vi "TPNT_CheckFileSize.vi"(8 "error in (no error)":errorcluster, 10 "maxfilesize":u32, 11 "File":path) -> (0 "error out":errorcluster, 2 "file moved":bool)   [LabVIEW 2016]
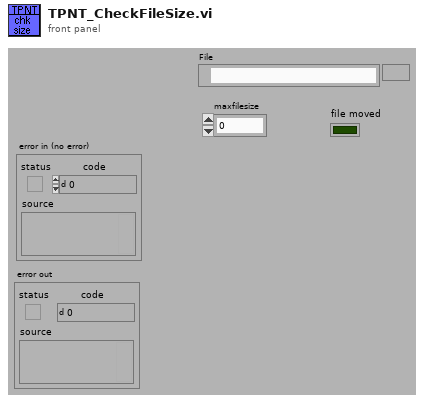
[diagram p1: front panel]
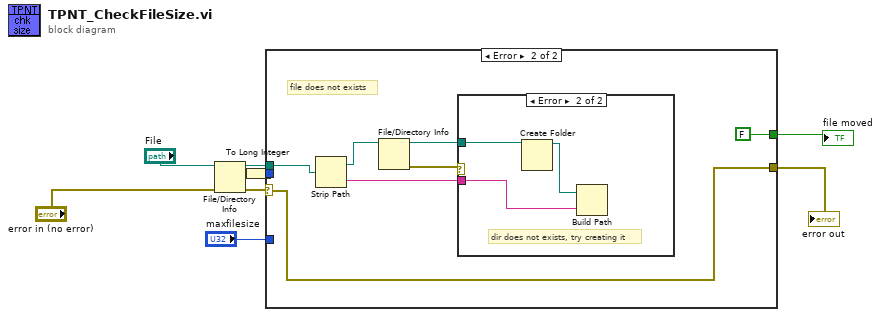
[diagram p0: block diagram]
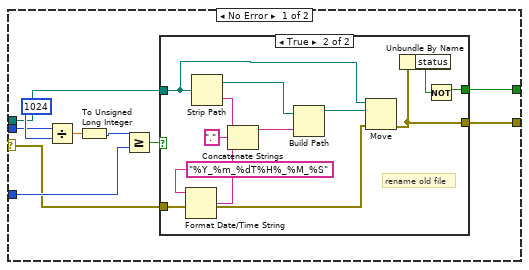
[diagram p2: hidden frame]
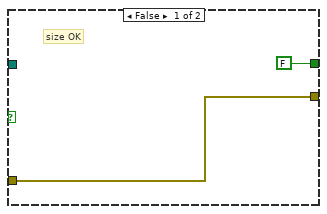
[diagram p3: hidden frame]
diagram:
  n1 = File/Directory Info(path="File", error in="error in (no error)") -> (path out=w5:path, size=w1:i64, error out=w4:errorcluster)  [unwired: 4 out]
  n2 = To Long Integer(number=w1) -> (32bit integer=w7:i32)
  n3 = case shown="Error" w4 {
    selector: w4 -> [w11 w34]
    tunnel: "maxfilesize" -> [w19 _]
    tunnel: w7 -> [w16 _]
    tunnel: w5 -> [w14 w39]
    tunnel: [w12 w34] -> w3
    tunnel: [w10 FALSE ("f")] -> w2
    frame No Error {
      n4 = Divide(x=w16, y=1024) -> (x/y=w17:dbl)
      n5 = To Unsigned Long Integer(number=w17) -> (unsigned 32bit integer=w15:u32)
      n6 = Greater Or Equal?(x=w15, y=w19) -> (x >= y?=w13:bool)
      n7 = case shown="True" w13 {
        tunnel: w14 -> [_ w26]
        tunnel: [w21 w24] -> w12
        tunnel: w11 -> [w21 w27]
        tunnel: [FALSE ("f") w22] -> w10
        frame False {
          # "size OK"
        }
        frame True {
          # "rename old file"
          n8 = Format Date/Time String(time format string (%c)="%Y_%m_%dT%H%_%M_%S") -> (date/time string=w30:string)  [unwired: 2 out]
          n9 = Strip Path(path=w26) -> (stripped path=w25:path, name=w33:string)
          n10 = Concatenate Strings(w33, "." ("string"), w30) -> (w29:string)
          n11 = Build Path(base path=w25, name or relative path=w29) -> (appended path=w28:path)
          n12 = Move(source path=w26, error in=w27, 10:w28) -> (error out=w24:errorcluster)  [unwired: 4 out]
          n13 = Unbundle By Name(w24) -> ("status"=w23:bool)
          n14 = Not(x=w23) -> (.not. x?=w22:bool)
        }
      }
    }
    frame Error {
      # "file does not exists"
      n15 = Strip Path(path=w39) -> (stripped path=w37:path, name=w38:string)
      n16 = File/Directory Info(path=w37) -> (path out=w35:path, error out=w36:errorcluster)  [unwired: 1 in, 5 out]
      n17 = case shown="Error" w36 {
        tunnel: w38 -> [_ w42]
        tunnel: w35 -> [_ w41]
        frame No Error {
          # "but directory does"
        }
        frame Error {
          # "dir does not exists, try creating it"
          n18 = Create Folder(path (use dialog)=w41) -> (created path=w43:path)  [unwired: 1 in, 3 out]
          n19 = Build Path(base path=w43, name or relative path=w42) -> ()  [unwired: 1 out]
        }
      }
    }
  }
  "error out" <- w3
  "file moved" <- w2
